vi "Chart.vi"() -> ()   [LabVIEW 2017, in "Chart.lvlib"]
uses:
  Chart.lvlib
  Communication/SubVIs/QueueRepo.Action.ctl
  Main/GUIReferences.Action.ctl
  <vilib>/Utility/miscctls.llb/LVPointTypeDef.ctl
  API/NewData.Data.ctl
  Communication/Communication.lvlib
  Main/MainGUI.lvlib
panel:
  out "Data":dbl[][](graph)
  in  "Rising?":bool=TRUE
  in  "Window Lenght":i32=10000 format="%.0p"
  in  "Trigger Signal":i32=1
  in  "Trigger Level":dbl=0.5
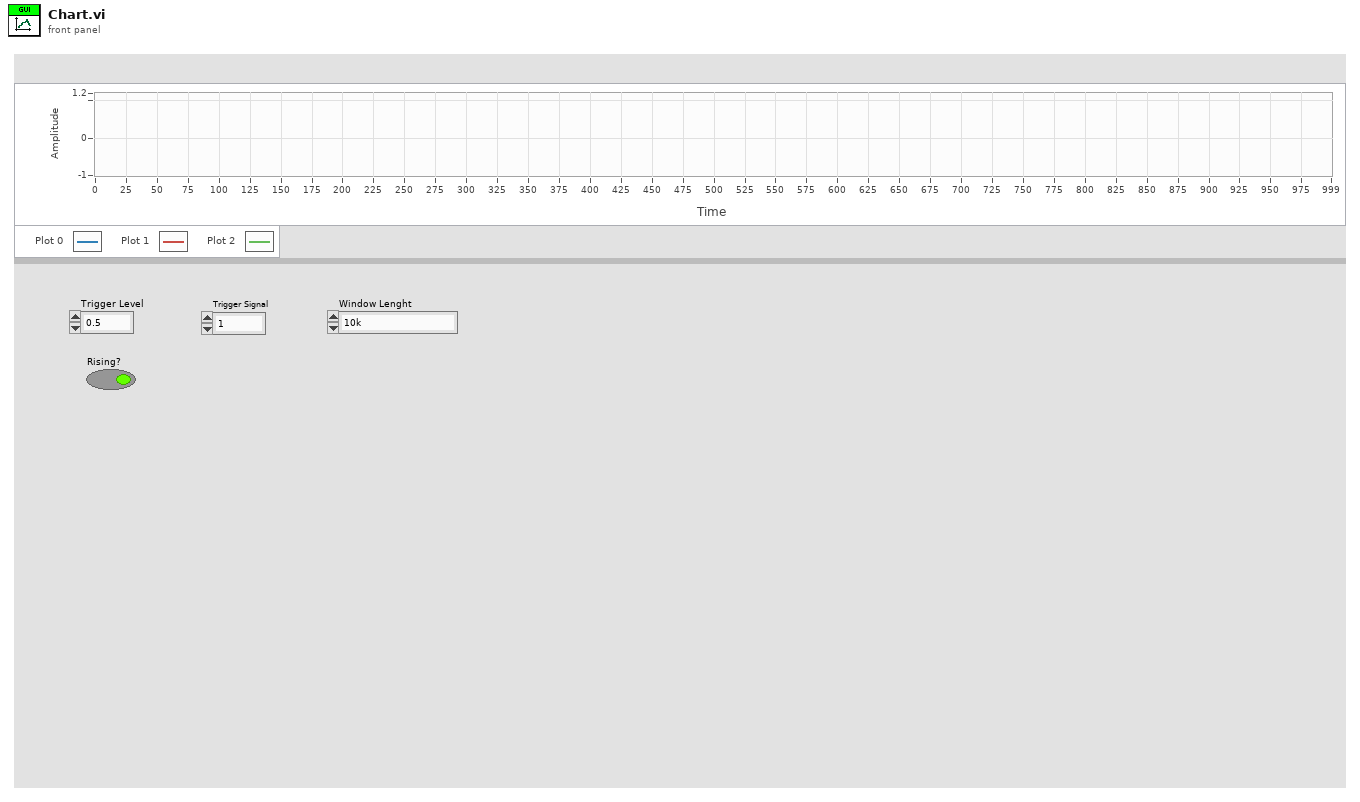
[diagram p1: front panel]
types:
  T1 = typedef "Communication.lvlib/QueueRepo.Action.ctl" = enum16{"Add", "Get", "Destroy", "Get All", "Clear"}
  T2 = typedef "MainGUI.lvlib/GUIReferences.Action.ctl" = enum16{"Get", "Register", "Unregister"}
  T3 = typedef "Chart.lvlib/NewData.Data.ctl" = cluster{"Data":dbl[][]}
  T4 = typedef "LVPointTypeDef.ctl" = cluster{"Horizontal":i16, "Vertical":i16}
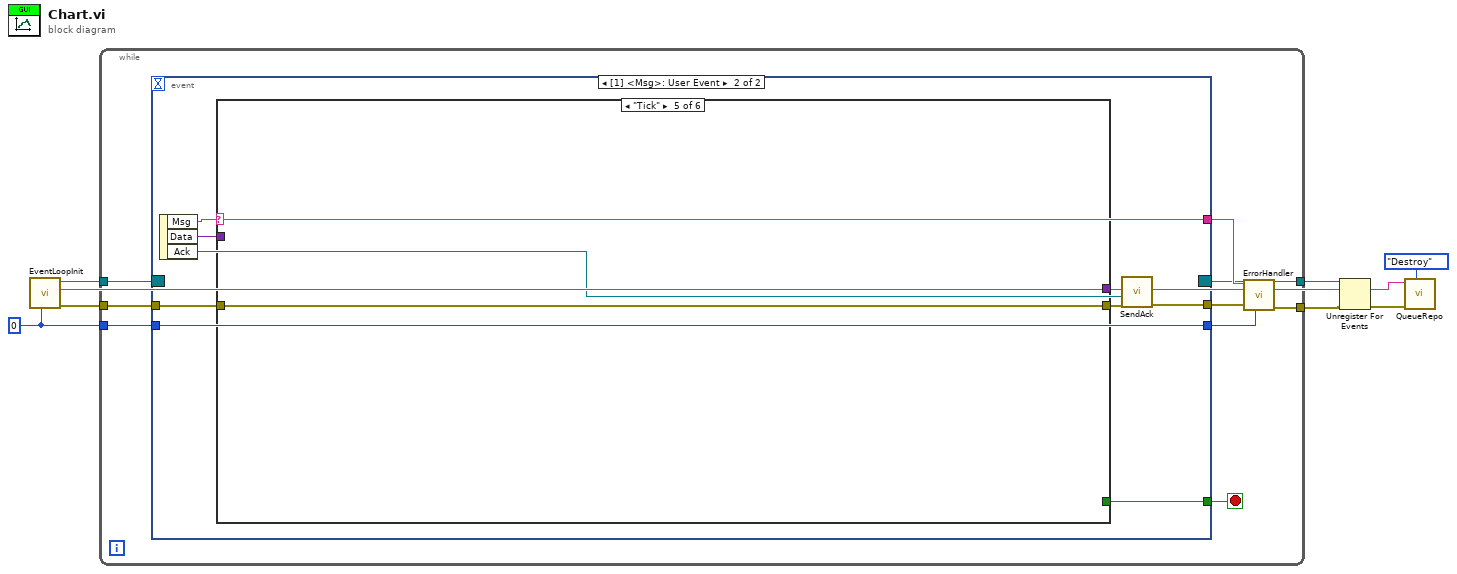
[diagram p0: block diagram]
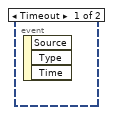
[diagram p2: hidden frame]
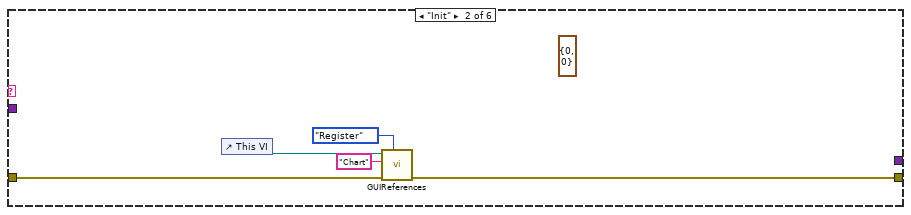
[diagram p4: hidden frame]
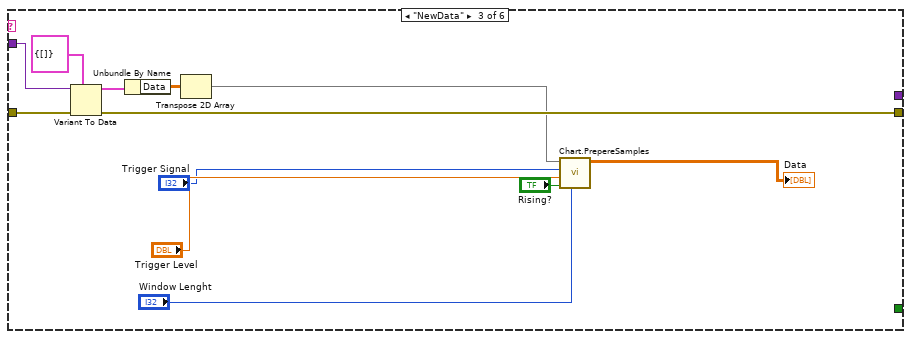
[diagram p5: hidden frame]
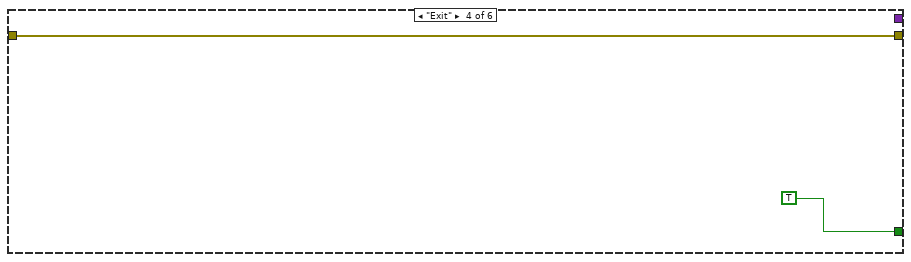
[diagram p6: hidden frame]
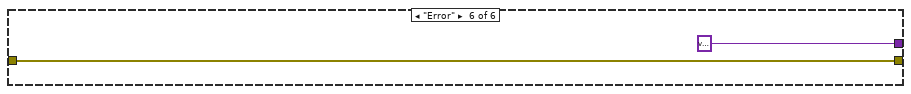
[diagram p7: hidden frame]
diagram:
  w6 = 0 ("Instance")
  n1 = call "EventLoopInit.vi"("Instance"=w6) -> ("error out"=w7:errorcluster, "Loop Name"=w5:string, "Event Registration Refnum"=w8:refnum<event-registration>)  [unwired: 8 in]
  n2 = while {
    tunnel: w8 -> [w17]
    tunnel: w7 -> [w16]
    tunnel: w6 -> [w15]
    tunnel: [w10] -> w2
    tunnel: [w9] -> w1
    stop <- w14 stop-if-true
    n3 = event shown="[1] <Msg>: User Event" {
      selector: w17 -> [_ _]
      dyn-events: [_ _] -> w10
      timeout: _ -> [_ _]
      tunnel: w16 -> [_ w25]
      tunnel: w15 -> [_ w19]
      tunnel: [_ w21] -> w14
      tunnel: [_ w20] -> w13
      tunnel: [_ w19] -> w12
      tunnel: [_ w18] -> w11
      event Timeout {
        n4 = event-data() -> ()  [unwired: 1 in, 3 out]
      }
      event User Event {
        n5 = event-data() -> ("Msg"=w18:string, "Data"=w26:variant, "Ack"=w24:refnum<notifier>)  [unwired: 1 in]
        n6 = case shown="\"Tick\"" w18 {
          tunnel: w26 -> [_ _ w42 _ _ _]
          tunnel: w25 -> [w27 w32 w44 w46 w47 w48]
          tunnel: [_ _ _ _ _ variant] -> w23
          tunnel: [w27 w31 w39 w46 w47 w48] -> w22
          tunnel: [_ _ _ TRUE _ _] -> w21
          frame Default {
          }
          frame "Init" {
            (unwired) T4 {"Horizontal"=0, "Vertical"=0} ("Origin")
            n7 = control-ref of="This VI"() -> (w28:refnum<vi>)
            n8 = call "GUIReferences.vi"("Action"=GUIReferences.Action."Register", "error in (no error)"=w32, "String"="Chart", "VI Refnum"=w28) -> ("error out"=w31:errorcluster)  [unwired: 6 in, 1 out]
          }
          frame "NewData" {
            n9 = Variant To Data(error in=w44, type=T3 {"Data"=[]} ("Cluster"), Variant=w42) -> (data=w41:T3, error out=w39:errorcluster)
            n10 = Unbundle By Name(w41) -> ("Data"=w40:dbl[][])
            n11 = Transpose 2D Array(2D array=w40) -> (transposed array=w34:dbl[][])
            n12 = call "Chart.PrepereSamples.vi"("Window Lenght"="Window Lenght", "Rising?"="Rising?", "Trigger Level"="Trigger Level", "Trigger Signal"="Trigger Signal", "Array in"=w34) -> ("Array out"=→"Data":dbl[][])  [unwired: 6 in]
          }
          frame "Exit" {
          }
          frame "Tick" {
          }
          frame "Error" {
          }
        }
        n13 = call "SendAck.vi"("error in (no error)"=w22, "Ack"=w24, "Variant"=w23) -> ("error out"=w20:errorcluster)  [unwired: 8 in]
      }
    }
    n14 = call "ErrorHandler.vi"("Instance"=w12, "error in (no error)"=w13, "Msg"=w11) -> ("error out"=w9:errorcluster)  [unwired: 8 in]
  }
  n15 = Unregister For Events(event registration refnum=w2, error in=w1) -> (error out=w4:errorcluster)
  n16 = call "QueueRepo.vi"("Action"=QueueRepo.Action."Destroy", "error in (no error)"=w4, "Name"=w5) -> ()  [unwired: 5 in, 4 out]
